vi "resultsInsertMessages.vi"(10 "chValuesIn":string[](array[string]), 11 "chNamesIn":string[](array[string])) -> (2 "chValuesOut":string[](array[string]), 3 "chNamesOut":string[](array[string]))   [LabVIEW 2020]
uses:
  Globals/Meas_global.vi
  Globals/Trav_pos_global.vi
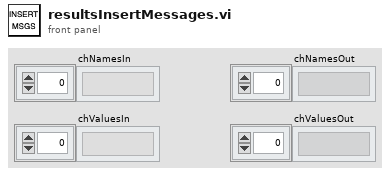
[diagram p1: front panel]
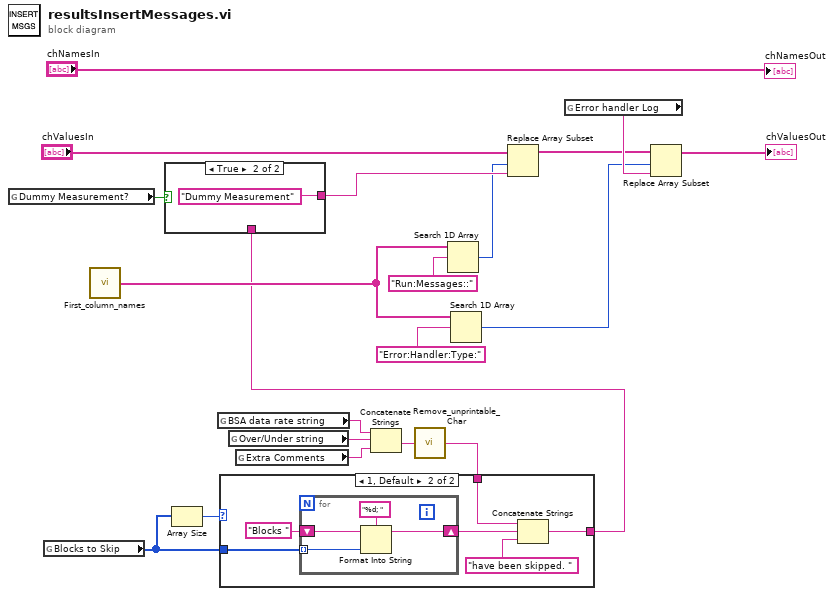
[diagram p0: block diagram]
diagram:
  n1 = global read "Trav_pos_global.vi" "Dummy Measurement?"() -> (w20:bool)
  n2 = global read "Meas_global.vi" "Blocks to Skip"() -> (w18:i32[])
  n3 = call "First_column_names.vi"() -> ("Array"=w19:string[])
  n4 = Array Size(array=w18) -> (size(s)=w16:i32)
  n5 = global read "Meas_global.vi" "BSA data rate string"() -> (w4:string)
  n6 = global read "Meas_global.vi" "Over/Under string"() -> (w2:string)
  n7 = global read "Meas_global.vi" "Extra Comments"() -> (w3:string)
  n8 = Concatenate Strings(w4, w2, w3) -> (w5:string)
  n9 = call "Remove_unprintable_Char.vi"("Input String"=w5) -> ("Output String"=w9:string)
  n10 = case shown="1, Default" w16 {
    tunnel: w18 -> [_ w27]
    tunnel: w9 -> [w21 w23]
    tunnel: [w21 w22] -> w10
    frame 0 {
    }
    frame 1, Default {
      n11 = for {
        shift-right: [w29] -> w25
        shift-left: "Blocks " -> [w31]
        tunnel: w27 -> [w30] mode=indexing
        n12 = Format Into String(format string="%d; ", initial string=w31, w30) -> (resulting string=w29:string)  [unwired: 1 in, 1 out]
      }
      n13 = Concatenate Strings(w23, w25, "have been skipped. " ("string")) -> (w22:string)
    }
  }
  n14 = case shown="True" w20 {
    tunnel: [w32 "Dummy Measurement"] -> w8
    tunnel: w10 -> [w32 _]
    frame False {
    }
    frame True {
    }
  }
  n15 = Search 1D Array(1D array=w19, element="Run:Messages::") -> (index of element=w6:i32)  [unwired: 1 out]
  n16 = Search 1D Array(1D array=w19, element="Error:Handler:Type:") -> (index of element=w13:i32)  [unwired: 1 out]
  n17 = Replace Array Subset(array="chValuesIn", new element=w8, index=w6) -> (w14:string[])
  n18 = global read "Meas_global.vi" "Error handler Log"() -> (w15:string)
  n19 = Replace Array Subset(array=w14, new element=w15, index=w13) -> (→"chValuesOut":string[])
  "chNamesOut" <- "chNamesIn"
